vi "Set Possible User Levels.vi"(0 "User Manager View in":refnum<class "User Manager View.lvclass">, 5 "User Level":T1, 11 "error in (no error)":errorcluster) -> (4 "User Manager View out":refnum<class "User Manager View.lvclass">, 15 "error out":errorcluster)   [LabVIEW 2017]
uses:
  User Manager View.lvclass
  User Manager Model/Type Definitions/User Levels.ctl
  User Manager Model/Type Definitions/User Manager Application Types.lvlib
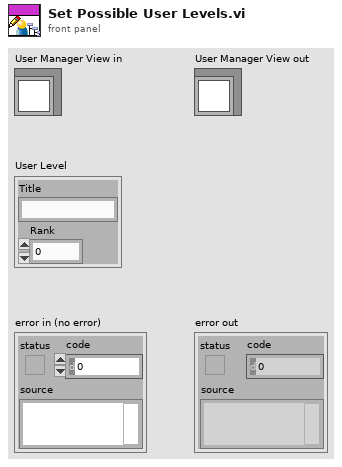
[diagram p1: front panel]
types:
  T1 = typedef "User Manager Application Types.lvlib/User Levels.ctl" = cluster{"Title":string, "Rank":i32}
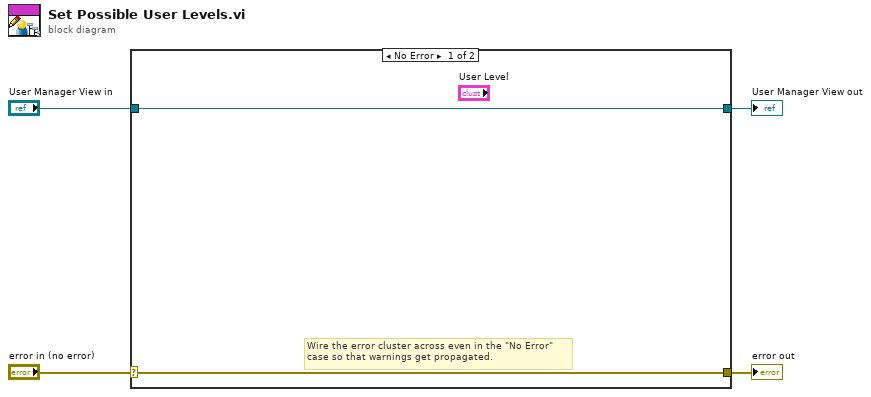
[diagram p0: block diagram]
diagram:
  n1 = case shown="No Error" "error in (no error)" {
    selector: "error in (no error)" -> [w5 w8]
    tunnel: [w5 w8] -> w3
    tunnel: [w6 w7] -> w1
    tunnel: "User Manager View in" -> [w6 w7]
    frame No Error {
      # "Wire the error cluster across even in the \"No Error\"\ncase so that warnings get propagated."
    }
    frame Error {
    }
  }
  "error out" <- w3
  "User Manager View out" <- w1
